vi "Check if bounding rectangle is in X & Y ranges.vi"(9 "Y range (pix)":cluster{"Min":i32, "Max":i32}={"Min"=50, "Max"=100}, 10 "Bounding Rect":T1={"Left"=10.0, "Top"=50.0, "Right"=20.0, "Bottom"=99.0}, 11 "X range (pix)":cluster{"Min":i32, "Max":i32}={"Min"=10, "Max"=20}) -> (2 "Rect in ranges?":bool=TRUE)   [LabVIEW 2013]
doc: "Checks if the input rectangle end pts are all inside the x and y ranges, if so set output to true."
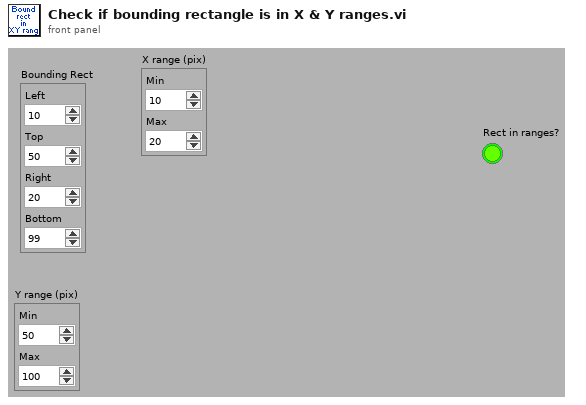
[diagram p1: front panel]
types:
  T1 = cluster{"Left":dbl, "Top":dbl, "Right":dbl, "Bottom":dbl}
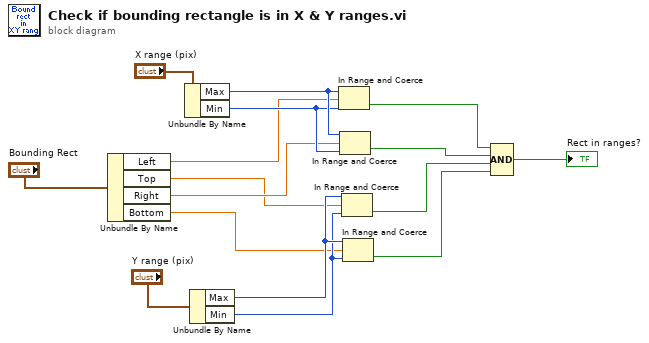
[diagram p0: block diagram]
diagram:
  n1 = Unbundle By Name("Bounding Rect") -> ("Left"=w9:dbl, "Top"=w7:dbl, "Right"=w8:dbl, "Bottom"=w6:dbl)
  n2 = Unbundle By Name("X range (pix)") -> ("Max"=w13:i32, "Min"=w12:i32)
  n3 = Unbundle By Name("Y range (pix)") -> ("Max"=w11:i32, "Min"=w10:i32)
  n4 = In Range and Coerce(upper limit=w13, x=w9, lower limit=w12) -> (In Range?=w5:bool)  [unwired: 1 out]
  n5 = In Range and Coerce(upper limit=w13, x=w8, lower limit=w12) -> (In Range?=w4:bool)  [unwired: 1 out]
  n6 = In Range and Coerce(upper limit=w11, x=w7, lower limit=w10) -> (In Range?=w3:bool)  [unwired: 1 out]
  n7 = In Range and Coerce(upper limit=w11, x=w6, lower limit=w10) -> (In Range?=w2:bool)  [unwired: 1 out]
  n8 = Compound Arithmetic op=AND(w5, w4, w3, w2) -> (→"Rect in ranges?":bool)
